vi "GT Arc YZC.vi"(0 "cardNum":i16, 1 "yCenter":dbl, 2 "circleDir":i16, 3 "synAcc":dbl, 5 "crd":i16, 7 "y":i32, 9 "z":i32, 10 "fifo":i16, 11 "error in (no error)":errorcluster caption="错误输入（无错误）", 12 "zCenter":dbl, 13 "synVel":dbl, 14 "velEnd":dbl) -> (4 "function return":i16, 15 "error out":errorcluster caption="错误输出")   [LabVIEW 2020, in "gts.lvlib"]
doc: "GT_API GT_ArcYZC(short cardNum,short crd,long y,long z,double yCenter,double zCenter,short circleDir,double synVel,double synAcc,double velEnd=0,short fifo=0);"
uses:
  gts.lvlib
  dll/32bit/multi_card/gts.dll
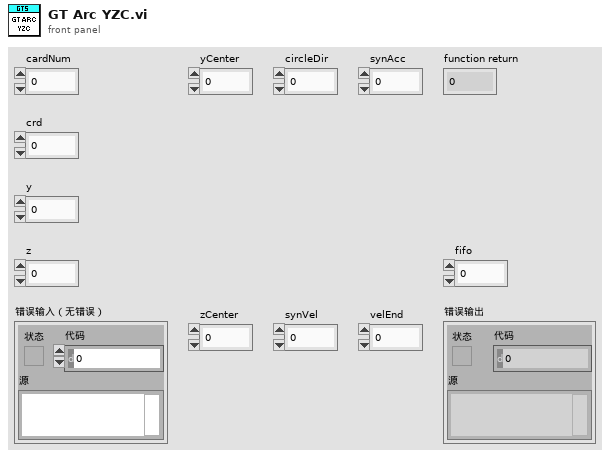
[diagram p1: front panel]
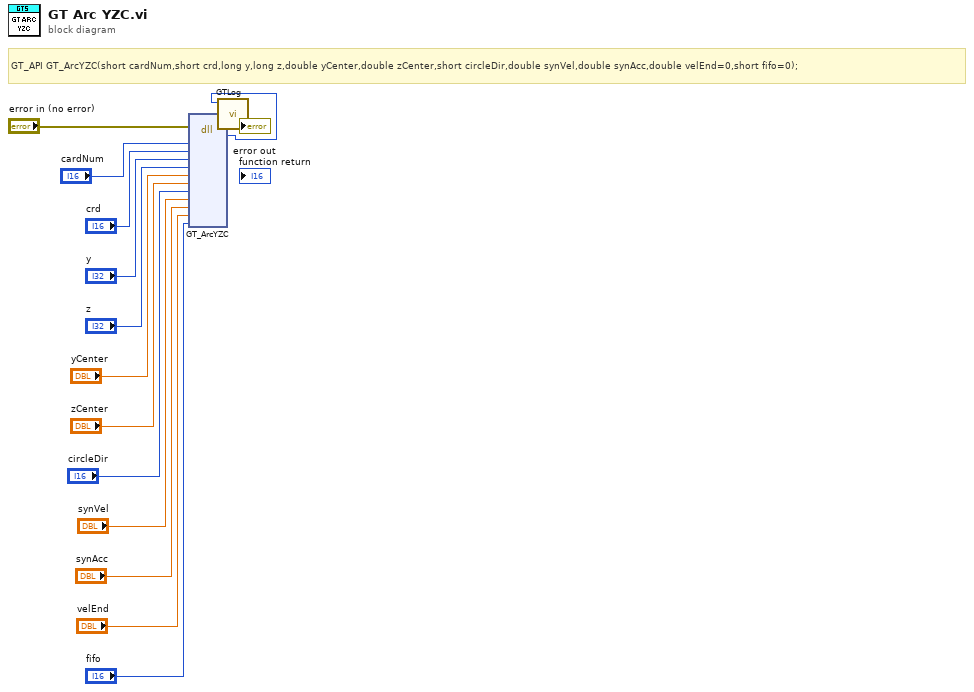
[diagram p0: block diagram]
diagram:
  # "GT_API GT_ArcYZC(short cardNum,short crd,long y,long z,double yCenter,double zCenter,short circleDir,double synVel,double synAcc,double velEnd=0,short fifo=0);"
  n1 = dll-call lib="C:/1228/dll/32bit/multi_card/gts.dll" fn="GT_ArcYZC"(error in="error in (no error)", "cardNum"="cardNum", "crd"="crd", "y"="y", "z"="z", "yCenter"="yCenter", "zCenter"="zCenter", "circleDir"="circleDir", "synVel"="synVel", "synAcc"="synAcc", "velEnd"="velEnd", "fifo"="fifo") -> (error out=w3:errorcluster, w1:i16)  [unwired: 13 in, 1 out]
  n2 = call "GTLog.vi"("error in (no error)"=w3, "Numeric"=w1) -> ("error out"=→"error out":errorcluster)  [unwired: 9 in]
